vi "Параллельный регистр.vi"(1 "C":bool, 2 "Reset":bool, 3 "Cluster":T2) -> (0 "output cluster":T1)   [LabVIEW 2013]
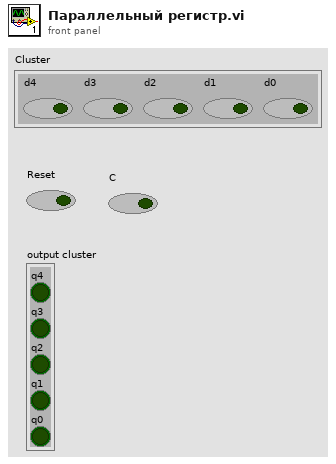
[diagram p1: front panel]
types:
  T1 = cluster{"q4":bool, "q3":bool, "q2":bool, "q1":bool, "q0":bool}
  T2 = cluster{"d4":bool, "d3":bool, "d2":bool, "d1":bool, "d0":bool}
  T3 = cluster{"q":bool, "q":bool, "q":bool, "q":bool, "q":bool}
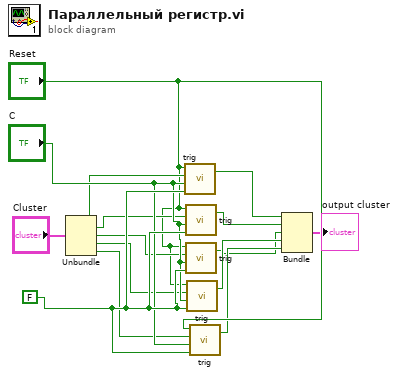
[diagram p0: block diagram]
diagram:
  w14 = FALSE
  n1 = Unbundle("Cluster") -> ("d4"=w8:bool, "d3"=w9:bool, "d2"=w10:bool, "d1"=w11:bool, "d0"=w12:bool)
  n2 = call "trig.vi"("s"=w14, "c"="C", "d"=w8, "r"="Reset") -> ("q"=w2:bool)  [unwired: 1 out]
  n3 = call "trig.vi"("s"=w14, "c"="C", "d"=w9, "r"="Reset") -> ("q"=w3:bool)  [unwired: 1 out]
  n4 = call "trig.vi"("s"=w14, "c"="C", "d"=w10, "r"="Reset") -> ("q"=w4:bool)  [unwired: 1 out]
  n5 = call "trig.vi"("s"=w14, "c"="C", "d"=w11, "r"="Reset") -> ("q"=w5:bool)  [unwired: 1 out]
  n6 = call "trig.vi"("s"=w14, "c"="C", "d"=w12, "r"="Reset") -> ("q"=w6:bool)  [unwired: 1 out]
  n7 = Bundle("q"=w2, "q"=w3, "q"=w4, "q"=w5, "q"=w6) -> (→"output cluster":T3)  [unwired: 1 in]
